vi "Registrar-Usuarios-V2.vi"() -> ()   [LabVIEW 2024]
uses:
  <vilib>/Utility/file.llb/Read Delimited Spreadsheet (string).vi
  <vilib>/Utility/file.llb/Write Delimited Spreadsheet (string).vi
panel:
  out "x = y?":bool
  in  "Tab Control":enum32{"Seleccionar ", "Registrar"}(tab)
  out "ActualUser":i32
  out "Array 2":i32[](array[numeric])
  out "Array":T1(array[cluster])
  out "Path":path=path "C:/Users/willi/GITHUB/TG/OBJ 2 - RECOLECCION DE DATOS/registro-usuarios.csv"
  out "Usserr":i32
  in  "Registrar Usuario":T2 {"Edad" format="%#_13g"}
  in  "registrButt":bool
  in  "stop":bool
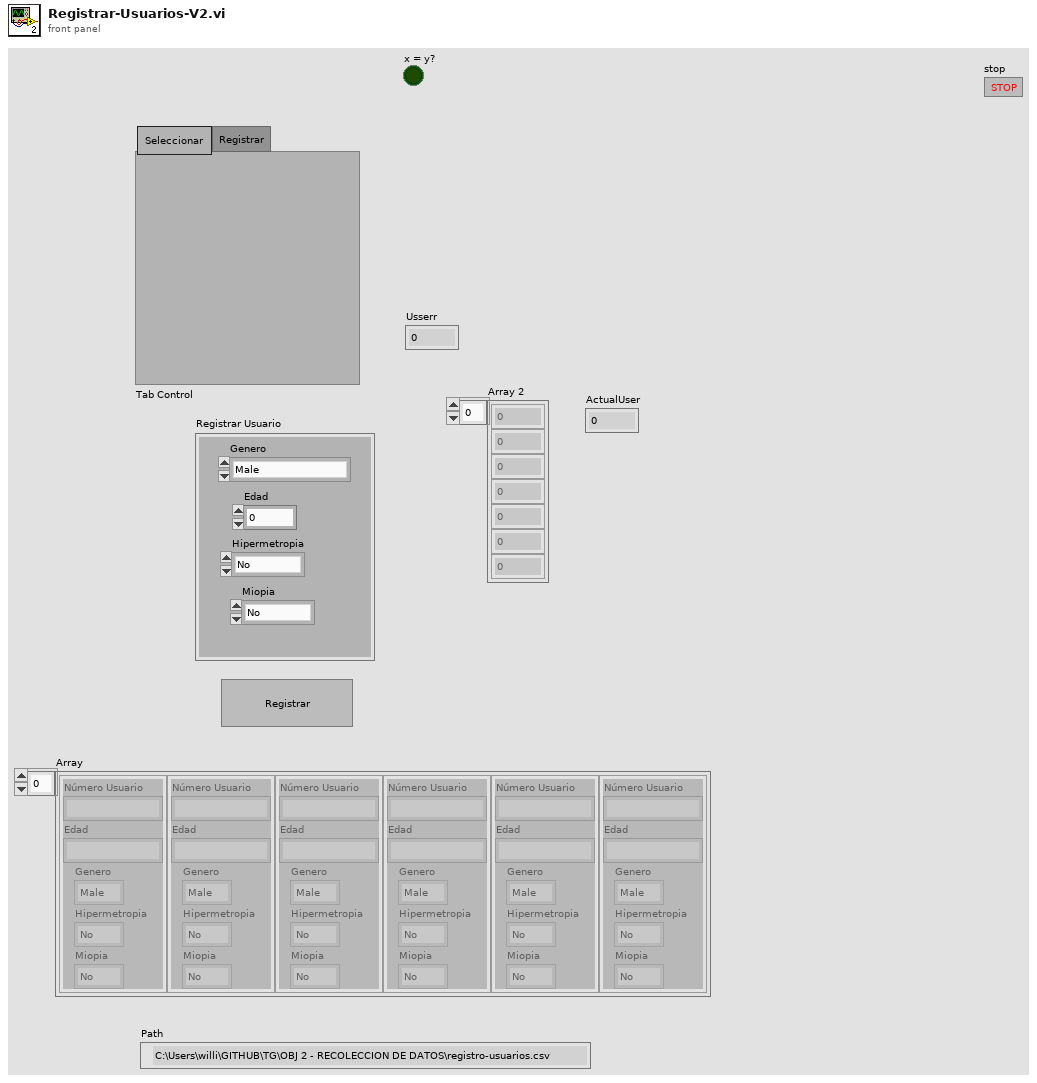
[diagram p1: front panel]
types:
  T1 = cluster{"Número Usuario":string, "Edad":string, "Genero":enum16{"Male", "Female"}, "Hipermetropia":enum16{"No", "Si"}, "Miopia":enum16{"No", "Si"}}[]
  T2 = cluster{"Genero":enum16{"Male", "Female"}, "Edad":dbl, "Hipermetropia":enum16{"No", "Si"}, "Miopia":enum16{"No", "Si"}}
  T3 = cluster{"Usuario":i32, "Genero":enum16{"Male", "Female"}, "Edad":dbl, "Hipermetropia":enum16{"No", "Si"}, "Miopia":enum16{"No", "Si"}}
  T4 = cluster{"Número Usuario":string, "Edad":string, "Genero":enum16{"Male", "Female"}, "Hipermetropia":enum16{"No", "Si"}, "Miopia":enum16{"No", "Si"}}
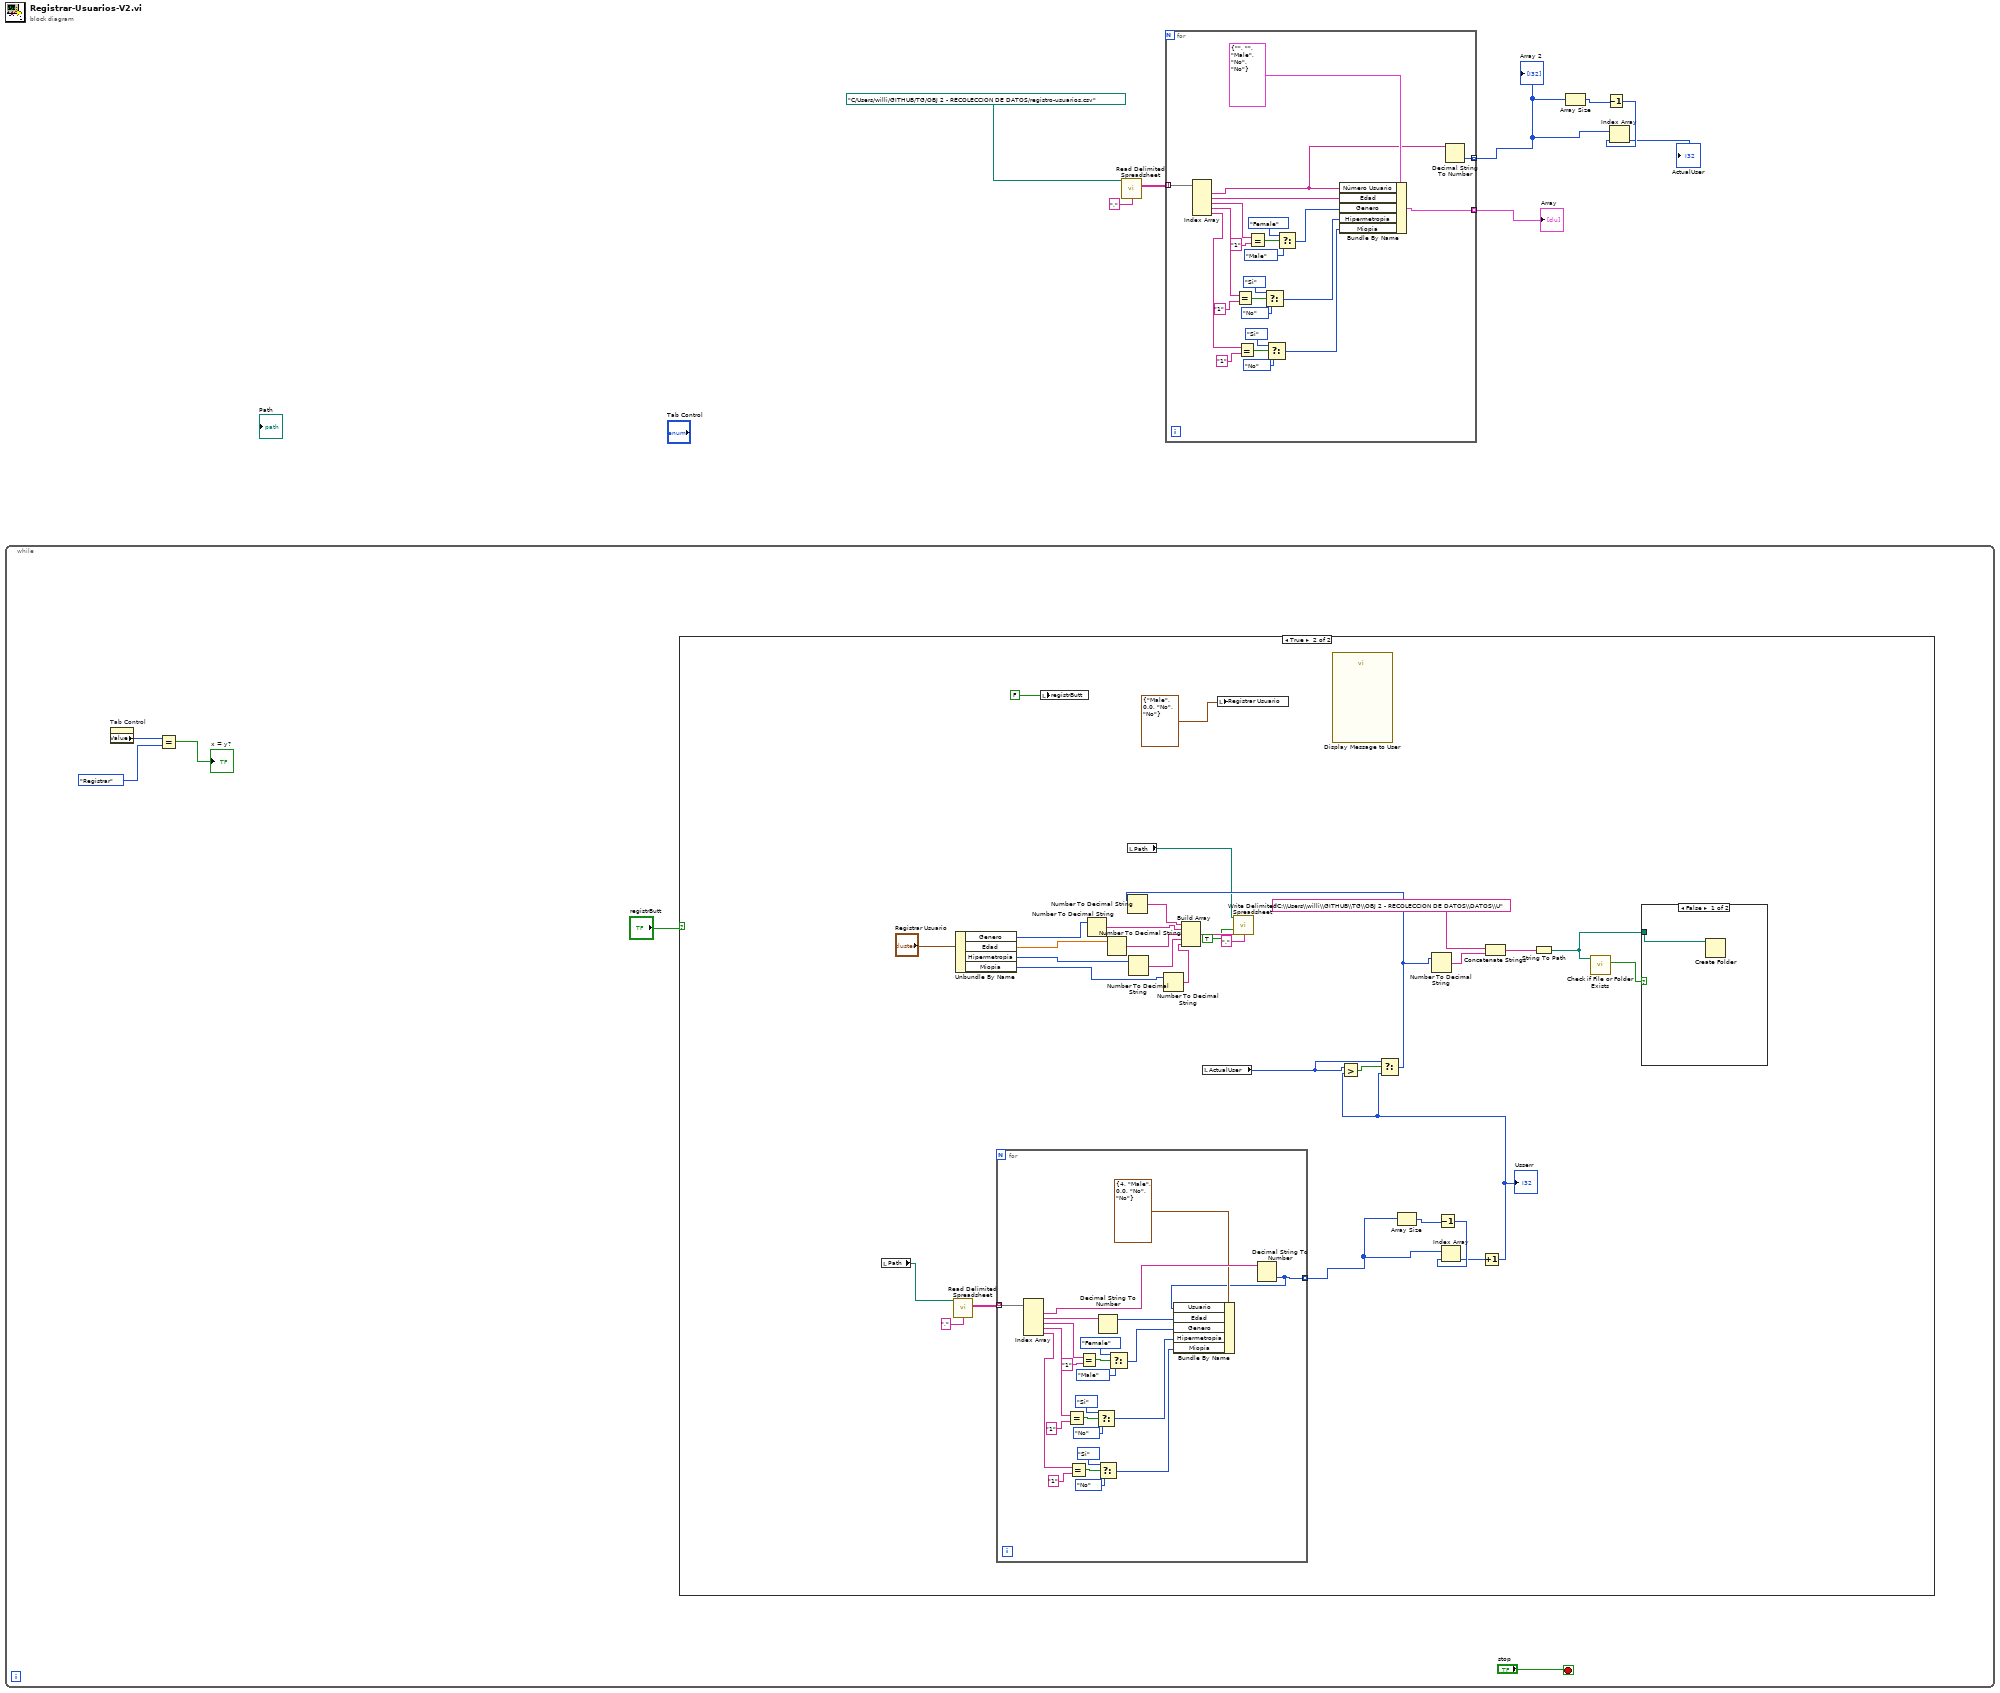
[diagram p0: block diagram]
diagram:
  n1 = while {
    stop <- "stop" stop-if-true
    n2 = property on="Tab Control" class="TabCtl (strict)"() -> ("Value"=w10:enum32{"Seleccionar ", "Registrar"})  [unwired: 2 in, 2 out]
    n3 = Equal?(x=w10, y=enum32{"Seleccionar ", "Registrar"}."Registrar" ("Tab Control")) -> (x = y?=→"x = y?":bool)
    n4 = case shown="True" "registrButt" {
      frame False {
      }
      frame True {
        n5 = local read "Path"() -> (w18:path)
        n6 = call-poly <vilib>:"Read Delimited Spreadsheet.vi"("file path (dialog if empty)"=w18, "delimiter (\\t)"="," ("delimiter (\\t)")) -> ("all rows"=w30:string[][])  [unwired: 8 in, 5 out]
        n7 = Unbundle By Name("Registrar Usuario") -> ("Genero"=w35:enum16{"Male", "Female"}, "Edad"=w34:dbl, "Hipermetropia"=w33:enum16{"No", "Si"}, "Miopia"=w32:enum16{"No", "Si"})
        n8 = for {
          tunnel: w30 -> [w70] mode=indexing
          tunnel: [w47] -> w29 mode=indexing
          n9 = Index Array(array=w70) -> (element #1=w51:string, element #2=w49:string, element #3=w68:string, element #4=w59:string, element #5=w53:string)  [unwired: 5 in]
          n10 = Equal?(x=w59, y="1") -> (x = y?=w62:bool)
          n11 = Equal?(x=w53, y="1") -> (x = y?=w56:bool)
          n12 = Equal?(x=w68, y="1") -> (x = y?=w67:bool)
          n13 = Select(t=enum16{"No", "Si"}."Si" ("Hipermetropia"), s=w62, f=enum16{"No", "Si"}."No" ("Hipermetropia")) -> (s? t:f=w58:enum16{"No", "Si"})
          n14 = Decimal String To Number(string=w49) -> (offset past number=w48:i32)  [unwired: 2 in, 1 out]
          n15 = Select(t=enum16{"No", "Si"}."Si" ("Hipermetropia"), s=w56, f=enum16{"No", "Si"}."No" ("Hipermetropia")) -> (s? t:f=w52:enum16{"No", "Si"})
          n16 = Select(t=enum16{"Male", "Female"}."Female" ("Genero"), s=w67, f=enum16{"Male", "Female"}."Male" ("Genero")) -> (s? t:f=w64:enum16{"Male", "Female"})
          n17 = Decimal String To Number(string=w51) -> (number=w47:i32)  [unwired: 2 in, 1 out]
          n18 = Bundle By Name(cluster=T3 {"Usuario"=4, "Genero"=enum."Male", "Edad"=0.0, "Hipermetropia"=enum."No", "Miopia"=enum."No"} ("Registrar Usuario"), "Usuario"=w47, "Edad"=w48, "Genero"=w64, "Hipermetropia"=w58, "Miopia"=w52) -> ()  [unwired: 1 out]
        }
        n19 = local write "registrButt"(FALSE) -> ()
        n20 = Number To Decimal String(number=w35) -> (decimal integer string=w36:string)  [unwired: 1 in]
        n21 = Number To Decimal String(number=w34) -> (decimal integer string=w39:string)  [unwired: 1 in]
        n22 = local read "Path"() -> (w17:path)
        n23 = Number To Decimal String(number=w33) -> (decimal integer string=w40:string)  [unwired: 1 in]
        n24 = Number To Decimal String(number=w32) -> (decimal integer string=w41:string)  [unwired: 1 in]
        n25 = local read "ActualUser"() -> (w23:i32)
        n26 = local write "Registrar Usuario"(T2 {"Genero"=enum."Male", "Edad"=0.0, "Hipermetropia"=enum."No", "Miopia"=enum."No"} ("Registrar Usuario")) -> ()
        n27 = call "Display Message to User"() -> ()  [unwired: 10 in, 2 out]
        n28 = Array Size(array=w29) -> (size(s)=w28:i32)
        n29 = Decrement(x=w28) -> (x-1=w27:i32)
        n30 = Index Array(array=w29, index=w27) -> (element=w26:i32)
        n31 = Increment(x=w26) -> (x+1=w22:i32)
        "Usserr" <- w22
        n32 = Greater?(x=w23, y=w22) -> (0:w24:bool)
        n33 = Select(t=w23, s=w24, f=w22) -> (s? t:f=w21:i32)
        n34 = Number To Decimal String(number=w21) -> (decimal integer string=w31:string)  [unwired: 1 in]
        n35 = Build Array(w31, w36, w39, w40, w41) -> (w44:string[])
        n36 = call-poly <vilib>:"Write Delimited Spreadsheet.vi"("file path (dialog if empty)"=w17, "1D data"=w44, "append to file? (new file:F)"=TRUE, "delimiter (\\t)"="," ("delimiter (\\t)")) -> ()  [unwired: 10 in, 2 out]
        n37 = Number To Decimal String(number=w21) -> (decimal integer string=w20:string)  [unwired: 1 in]
        n38 = Concatenate Strings("C:\\Users\\willi\\GITHUB\\TG\\OBJ 2 - RECOLECCION DE DATOS\\DATOS\\U" ("string"), w20) -> (w16:string)
        n39 = String To Path(string=w16) -> (path=w14:path)
        n40 = call <vilib>:"Check if File or Folder Exists.vi"("path"=w14) -> ("file or folder exists?"=w15:bool)  [unwired: 8 in, 2 out]
        n41 = case shown="False" w15 {
          tunnel: w14 -> [w46 _]
          frame False {
            n42 = Create Folder(path (use dialog)=w46) -> ()  [unwired: 2 in, 3 out]
          }
          frame True {
          }
        }
      }
    }
  }
  n43 = call-poly <vilib>:"Read Delimited Spreadsheet.vi"("file path (dialog if empty)"=path "C:/Users/willi/GITHUB/TG/OBJ 2 - RECOLECCION DE DATOS/registro-usuarios.csv", "delimiter (\\t)"="," ("delimiter (\\t)")) -> ("all rows"=w7:string[][])  [unwired: 8 in, 5 out]
  n44 = for {
    tunnel: w7 -> [w94] mode=indexing
    tunnel: [w73] -> w6 mode=indexing
    tunnel: [w71] -> w4 mode=indexing
    n45 = Index Array(array=w94) -> (element #1=w72:string, element #2=w92:string, element #3=w90:string, element #4=w81:string, element #5=w75:string)  [unwired: 5 in]
    n46 = Equal?(x=w81, y="1") -> (x = y?=w84:bool)
    n47 = Equal?(x=w75, y="1") -> (x = y?=w78:bool)
    n48 = Equal?(x=w90, y="1") -> (x = y?=w89:bool)
    n49 = Select(t=enum16{"No", "Si"}."Si" ("Hipermetropia"), s=w84, f=enum16{"No", "Si"}."No" ("Hipermetropia")) -> (s? t:f=w80:enum16{"No", "Si"})
    n50 = Select(t=enum16{"No", "Si"}."Si" ("Hipermetropia"), s=w78, f=enum16{"No", "Si"}."No" ("Hipermetropia")) -> (s? t:f=w74:enum16{"No", "Si"})
    n51 = Select(t=enum16{"Male", "Female"}."Female" ("Genero"), s=w89, f=enum16{"Male", "Female"}."Male" ("Genero")) -> (s? t:f=w86:enum16{"Male", "Female"})
    n52 = Bundle By Name(cluster=T4 {"Número Usuario"="", "Edad"="", "Genero"=enum."Male", "Hipermetropia"=enum."No", "Miopia"=enum."No"} ("Registrar Usuario"), "Número Usuario"=w72, "Edad"=w92, "Genero"=w86, "Hipermetropia"=w80, "Miopia"=w74) -> (w73:T4)
    n53 = Decimal String To Number(string=w72) -> (number=w71:i32)  [unwired: 2 in, 1 out]
  }
  "Array" <- w6
  "Array 2" <- w4
  n54 = Array Size(array=w4) -> (size(s)=w3:i32)
  n55 = Decrement(x=w3) -> (x-1=w2:i32)
  n56 = Index Array(array=w4, index=w2) -> (element=→"ActualUser":i32)
